vi "ep_Check Wiring Error.vi"(7 "reset? (F)":bool, 8 "error in (no error)":errorcluster, 9 "system info in":refnum<class "EP System Info.lvclass">, 10 "physical channels in":T1[](array[typedef])=[enum."Voltage Phase A (L1)", enum."Voltage Phase B (L2)", enum."Voltage Phase C (L3)", enum."Current Phase A (L1)", enum."Current Phase B (L2)", enum."Current Phase C (L3)", enum."Current Phase N (Neutral)"], 11 "data in":sgl[][](array[numeric]) format="%#.21g") -> (0 "error out":errorcluster, 1 "system info out":refnum<class "EP System Info.lvclass">, 2 "physical channels out":T1[](array[typedef])=[enum."Voltage Phase A (L1)", enum."Voltage Phase B (L2)", enum."Voltage Phase C (L3)", enum."Current Phase A (L1)", enum."Current Phase B (L2)", enum."Current Phase C (L3)", enum."Current Phase N (Neutral)"], 3 "data out":sgl[][](array[numeric]) format="%#.21g")   [LabVIEW 2011, in "NI_EP_Power Quality.lvlib"]
uses:
  <vilib>/addons/Electrical Power/PQ/NI_EP_Power Quality.lvlib
  <vilib>/addons/Electrical Power/PQ/Common/Controls/ep_AI Data Channel.ctl
  <vilib>/addons/Electrical Power/PQ/Common/Classes/System Info/EP System Info.lvclass
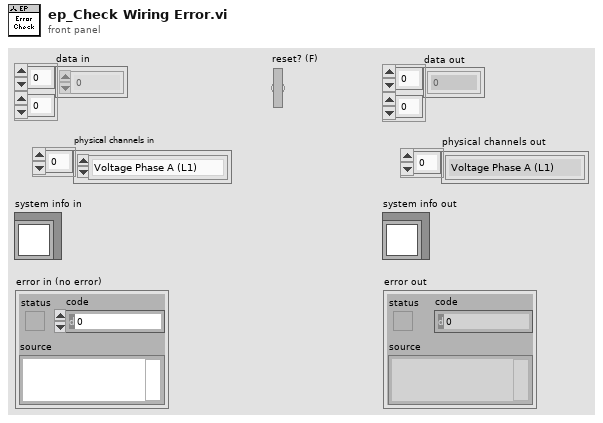
[diagram p1: front panel]
types:
  T1 = typedef "NI_EP_Power Quality.lvlib/ep_AI Data Channel.ctl" = enum16{"Voltage Phase A (L1)", "Voltage Phase B (L2)", "Voltage Phase C (L3)", "Voltage Phase N (Neutral)", "Current Phase A (L1)", "Current Phase B (L2)", "Current Phase C (L3)", "Current Phase N (Neutral)"}
  T2 = typedef "NI_EP_Power Quality.lvlib/ep_Wiring.ctl" = enum16{"4xUph + 4xI", "3xUph + 4xI", "3xUline + 4xI", "3xUph + 3xI", "3xUline + 3xI", "3xUph + 2xI", "3xUline + 2xI", "1xUph + 1xI"}
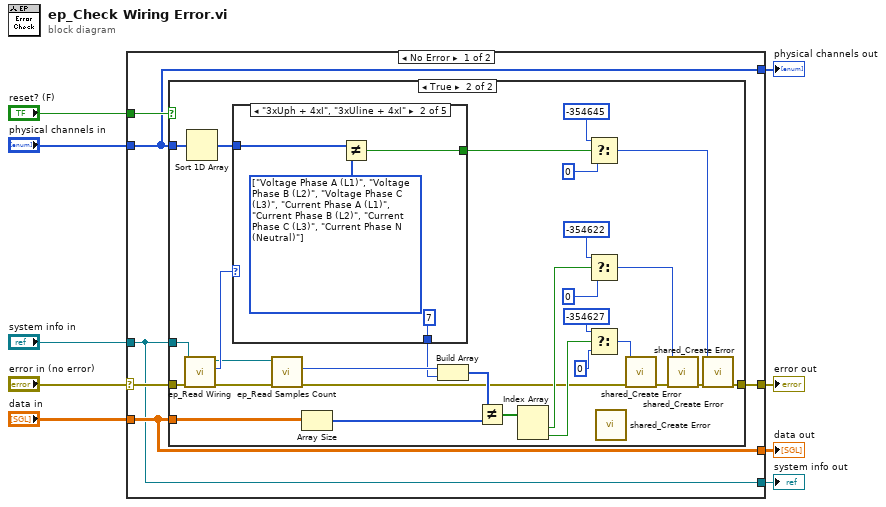
[diagram p0: block diagram]
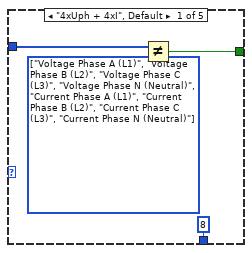
[diagram p3: hidden frame]
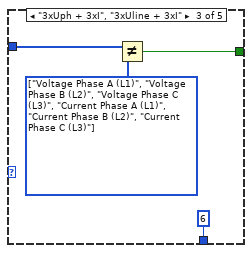
[diagram p4: hidden frame]
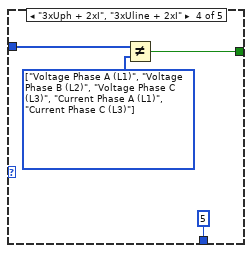
[diagram p5: hidden frame]
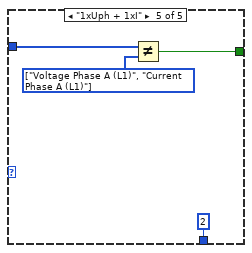
[diagram p6: hidden frame]
diagram:
  n1 = case shown="No Error" "error in (no error)" {
    selector: "error in (no error)" -> [w15 w67]
    tunnel: "system info in" -> [w10 w66]
    tunnel: "reset? (F)" -> [w14 _]
    tunnel: "physical channels in" -> [w12 _]
    tunnel: "data in" -> [w11 _]
    tunnel: [w13 w67] -> w4
    tunnel: [w12 _] -> w3
    tunnel: [w11 _] -> w2
    tunnel: [w10 w66] -> w1
    frame No Error {
      n2 = case shown="True" w14 {
        tunnel: w15 -> [w16 w45]
        tunnel: w10 -> [_ w44]
        tunnel: w12 -> [_ w43]
        tunnel: w11 -> [_ w36]
        tunnel: [w16 w27] -> w13
        frame False {
        }
        frame True {
          n3 = call <vilib>:"ep_Read Wiring.vi"("error in (no error)"=w45, "system info in"=w44) -> ("error out"=w37:errorcluster, "wiring"=w42:T2, "system info out"=w38:refnum<class "EP System Info.lvclass">)  [unwired: 6 in, 1 out]
          n4 = Sort 1D Array(array=w43) -> (sorted array=w41:T1[])
          n5 = case shown="\"3xUph + 4xI\", \"3xUline + 4xI\"" w42 {
            tunnel: w41 -> [w49 w53 w57 w61 w64]
            tunnel: [w47 w51 w55 w58 w62] -> w28
            tunnel: [8 ("element") 7 ("element") 6 ("element") 5 ("element") 2 ("element")] -> w32
            frame "4xUph + 4xI", Default {
              w48 = T1[] [enum."Voltage Phase A (L1)", enum."Voltage Phase B (L2)", enum."Voltage Phase C (L3)", enum."Voltage Phase N (Neutral)", enum."Current Phase A (L1)", enum."Current Phase B (L2)", enum."Current Phase C (L3)", enum."Current Phase N (Neutral)"] items=["Voltage Phase A (L1)", "Voltage Phase B (L2)", "Voltage Phase C (L3)", "Voltage Phase N (Neutral)", "Current Phase A (L1)", "Current Phase B (L2)", "Current Phase C (L3)", "Current Phase N (Neutral)"] ("physical channels")
              n6 = Not Equal?(x=w49, y=w48) -> (x != y?=w47:bool)
            }
            frame "3xUph + 4xI", "3xUline + 4xI" {
              w52 = T1[] [enum."Voltage Phase A (L1)", enum."Voltage Phase B (L2)", enum."Voltage Phase C (L3)", enum."Current Phase A (L1)", enum."Current Phase B (L2)", enum."Current Phase C (L3)", enum."Current Phase N (Neutral)"] items=["Voltage Phase A (L1)", "Voltage Phase B (L2)", "Voltage Phase C (L3)", "Voltage Phase N (Neutral)", "Current Phase A (L1)", "Current Phase B (L2)", "Current Phase C (L3)", "Current Phase N (Neutral)"] ("physical channels")
              n7 = Not Equal?(x=w53, y=w52) -> (x != y?=w51:bool)
            }
            frame "3xUph + 3xI", "3xUline + 3xI" {
              w56 = T1[] [enum."Voltage Phase A (L1)", enum."Voltage Phase B (L2)", enum."Voltage Phase C (L3)", enum."Current Phase A (L1)", enum."Current Phase B (L2)", enum."Current Phase C (L3)"] items=["Voltage Phase A (L1)", "Voltage Phase B (L2)", "Voltage Phase C (L3)", "Voltage Phase N (Neutral)", "Current Phase A (L1)", "Current Phase B (L2)", "Current Phase C (L3)", "Current Phase N (Neutral)"] ("physical channels")
              n8 = Not Equal?(x=w57, y=w56) -> (x != y?=w55:bool)
            }
            frame "3xUph + 2xI", "3xUline + 2xI" {
              w60 = T1[] [enum."Voltage Phase A (L1)", enum."Voltage Phase B (L2)", enum."Voltage Phase C (L3)", enum."Current Phase A (L1)", enum."Current Phase C (L3)"] items=["Voltage Phase A (L1)", "Voltage Phase B (L2)", "Voltage Phase C (L3)", "Voltage Phase N (Neutral)", "Current Phase A (L1)", "Current Phase B (L2)", "Current Phase C (L3)", "Current Phase N (Neutral)"] ("physical channels")
              n9 = Not Equal?(x=w61, y=w60) -> (x != y?=w58:bool)
            }
            frame "1xUph + 1xI" {
              w65 = T1[] [enum."Voltage Phase A (L1)", enum."Current Phase A (L1)"] items=["Voltage Phase A (L1)", "Voltage Phase B (L2)", "Voltage Phase C (L3)", "Voltage Phase N (Neutral)", "Current Phase A (L1)", "Current Phase B (L2)", "Current Phase C (L3)", "Current Phase N (Neutral)"] ("physical channels")
              n10 = Not Equal?(x=w64, y=w65) -> (x != y?=w62:bool)
            }
          }
          n11 = call <vilib>:"ep_Read Samples Count.vi"("error in (no error)"=w37, "system info in"=w38) -> ("error out"=w19:errorcluster, "basic calc. interval (samples)"=w35:i32)  [unwired: 5 in, 3 out]
          n12 = Array Size(array=w36) -> (size(s)=w34:i32[])
          n13 = Build Array(w35, w32) -> (w33:i32[])
          n14 = Not Equal?(x=w33, y=w34) -> (x != y?=w24:bool[])
          n15 = Index Array(array=w24) -> (element #1=w23:bool, element #2=w22:bool)  [unwired: 2 in]
          n16 = Select(t=-354645, s=w28, f=0 ("error code (0)")) -> (s? t:f=w39:i32)
          n17 = Select(t=-354622, s=w23, f=0 ("error code (0)")) -> (s? t:f=w30:i32)
          n18 = Select(t=-354627, s=w22, f=0) -> (s? t:f=w17:i32)
          n19 = call <vilib>:"shared_Create Error.vi"() -> ()  [unwired: 11 in, 1 out]
          n20 = call <vilib>:"shared_Create Error.vi"("error in (no error)"=w19, "error code (0)"=w17) -> ("error out"=w18:errorcluster)  [unwired: 9 in]
          n21 = call <vilib>:"shared_Create Error.vi"("error in (no error)"=w18, "error code (0)"=w30) -> ("error out"=w29:errorcluster)  [unwired: 9 in]
          n22 = call <vilib>:"shared_Create Error.vi"("error in (no error)"=w29, "error code (0)"=w39) -> ("error out"=w27:errorcluster)  [unwired: 9 in]
        }
      }
    }
    frame Error {
    }
  }
  "error out" <- w4
  "data out" <- w2
  "physical channels out" <- w3
  "system info out" <- w1
